vi "Actor Core.vi"(8 "error in":errorcluster, 11 "SensorCharm in":refnum<class "SensorCharm.lvclass">) -> (0 "error out":errorcluster, 3 "Actor out":refnum<class "Actor.lvclass">)   [LabVIEW 2012, in "Sensor Definition.lvlib" / "SensorCharm.lvclass"]
doc: "(<B>Filename</B>: Actor Framework.lvlib:Actor.lvclass:Actor Core.vi)\n\nReceives messages to the actor, reacts to them, and initiates any error handling that may shut the actor down.\n\nDescendant classes may override this VI to append parallel tasks for the actor to complete while it handles messages. Overrides use the Call Parent Method node."
uses:
  SensorCharm.lvclass
  <vilib>/ActorFramework/Actor/Actor.lvclass
  Controls/String XControl/String XControl.xctl
  Win8uiFramework/CharmView.lvclass
  <vilib>/ActorFramework/Actor/Actor.lvclass/Actor.ctl
  <vilib>/ActorFramework/Message Enqueuer/Message Enqueuer.lvclass/Message Enqueuer.ctl
  Win8uiFramework/ViewableActor.lvclass/ViewableActor.ctl
  SensorCharm.lvclass/SensorCharm.ctl
  SensorInfo.lvclass/SensorInfo.ctl
  Sensor Messages/Update Sensor Info and Re-broadcast Msg/Update Sensor Info and Re-broadcast Msg.lvclass/Update Sensor Info and Re-broadcast Msg.ctl
  SensorInfo/Write Name.vi
  Write Description.vi
  SensorInfo/Write Sample Time.vi
  Win8uiFramework/Read Stop Event.vi
  Read SensorInfo.vi
  SensorInfo/Read Name.vi
  SensorInfo/Read Description.vi
  SensorInfo/Read Sample Time.vi
  <vilib>/ActorFramework/Message Enqueuer/Init from Existing Queue.vi
  <vilib>/ActorFramework/Message Enqueuer/Enqueue.vi
  <vilib>/ActorFramework/Message Priority Queue/Priority Enqueue.vi
  <vilib>/ActorFramework/Message Enqueuer/Message Enqueuer.lvclass
  SensorInfo.lvclass
  Sensor Messages/Update Sensor Info and Re-broadcast Msg/Update Sensor Info and Re-broadcast Msg.lvclass
  Win8uiFramework/ViewableActor.lvclass
panel:
  in  "Name String":string="Name"
  in  "Sample Period (s)":dbl=0.5
  in  "Description String":string="Description of what and/or where this sensor is."
  out "Title":string(xcontrol)
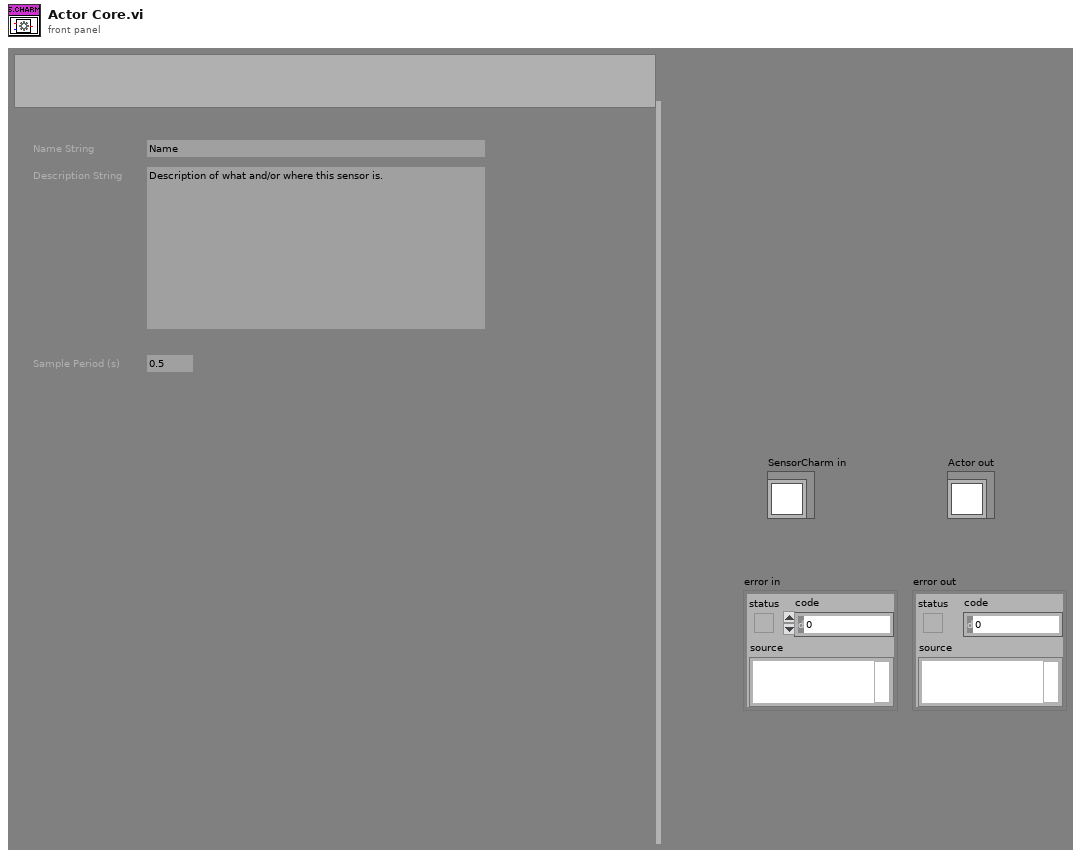
[diagram p1: front panel]
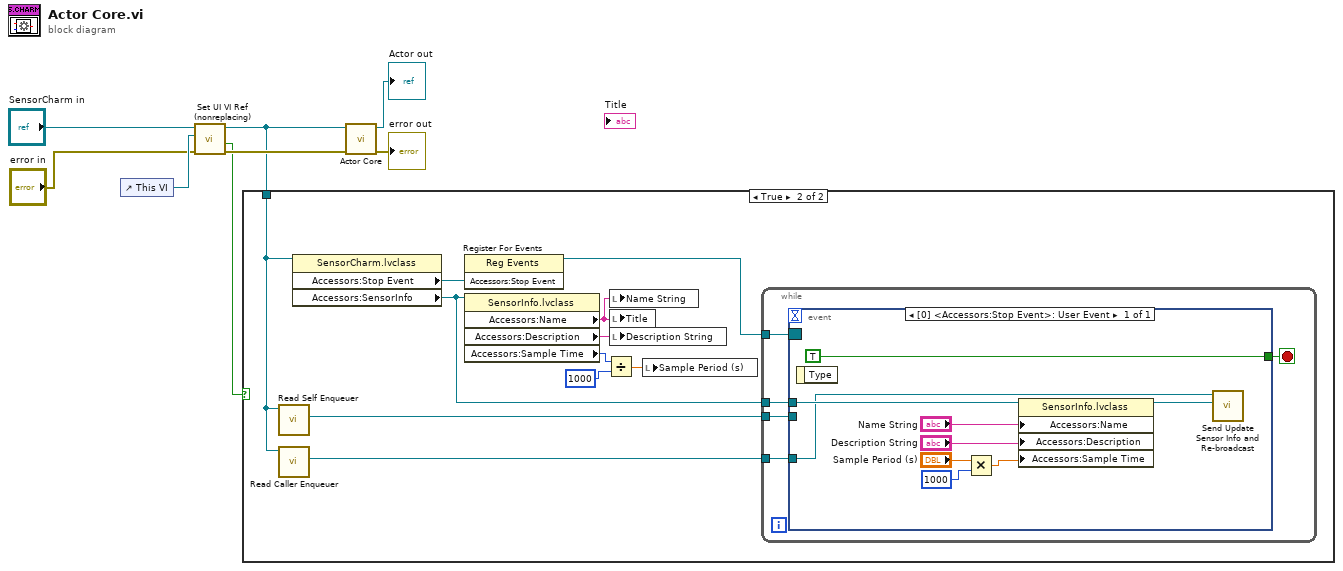
[diagram p0: block diagram]
diagram:
  n1 = control-ref of="This VI"() -> (w6:refnum<vi>)
  n2 = call "Set UI VI Ref (nonreplacing).vi"("error in (no error)"="error in", "UI VI Ref"=w6, "ViewableActor in"="SensorCharm in") -> ("error out"=w3:errorcluster, "Top Level UI?"=w2:bool, "ViewableActor out"=w1:refnum<class "SensorCharm.lvclass">)  [unwired: 6 in]
  n3 = case shown="True" w2 {
    tunnel: w1 -> [_ w16]
    frame False {
    }
    frame True {
      n4 = call <vilib>:"Read Self Enqueuer.vi"("Actor"=w16) -> ("Self Enqueuer"=w17:refnum<class "Message Enqueuer.lvclass">)  [unwired: 10 in]
      n5 = call <vilib>:"Read Caller Enqueuer.vi"("Actor"=w16) -> ("Caller Enqueuer"=w15:refnum<class "Message Enqueuer.lvclass">)  [unwired: 10 in]
      n6 = property class="SensorCharm.lvclass"(reference=w16) -> ("Accessors:Stop Event"=w19:refnum<user-event>, "Accessors:SensorInfo"=w12:refnum<class "SensorInfo.lvclass">)  [unwired: 1 in, 2 out]
      n7 = register-events(w19) -> (reference out=w18:refnum<event-registration>)  [unwired: 2 in, 1 out]
      n8 = property class="SensorInfo.lvclass"(reference=w12) -> ("Accessors:Name"=w14:string, "Accessors:Description"=w13:string, "Accessors:Sample Time"=w11:i32)  [unwired: 1 in, 2 out]
      n9 = Divide(x=w11, y=1000) -> (x/y=w9:dbl)
      n10 = local write "Name String"(w14) -> ()
      n11 = local write "Title"(w14) -> ()
      n12 = local write "Description String"(w13) -> ()
      n13 = local write "Sample Period (s)"(w9) -> ()
      n14 = while {
        tunnel: w18 -> [w24]
        tunnel: w17 -> [w22]
        tunnel: w15 -> [w21]
        tunnel: w12 -> [w20]
        stop <- w23 stop-if-true
        n15 = event shown="[0] <Accessors:Stop Event>: User Event" {
          selector: w24 -> [_]
          dyn-events: _ -> [_]
          timeout: _ -> [_]
          tunnel: [TRUE] -> w23
          tunnel: w22 -> [_]
          tunnel: w21 -> [w25]
          tunnel: w20 -> [w32]
          event User Event {
            n16 = event-data() -> ()  [unwired: 1 in, 1 out]
            n17 = Multiply(x="Sample Period (s)", y=1000) -> (x*y=w26:dbl)
            n18 = property class="SensorInfo.lvclass"(reference=w32, "Accessors:Name"="Name String", "Accessors:Description"="Description String", "Accessors:Sample Time"=w26) -> (reference out=w29:refnum<class "SensorInfo.lvclass">)  [unwired: 1 in, 1 out]
            n19 = call "Send Update Sensor Info and Re-broadcast.vi"("SensorInfo"=w29, "Message Enqueuer"=w25) -> ()  [unwired: 8 in, 2 out]
          }
        }
      }
    }
  }
  n20 = call-parent "Actor Core.vi"("error in"=w3, "CharmView in"=w1) -> ("error out"=→"error out":errorcluster, "Actor out"=→"Actor out":refnum<class "Actor.lvclass">)  [unwired: 8 in]
